vi "Tx Status to DBLs.vi"(3 "TxStatus":T1) -> (1 "TxStatusDBLs":dbl[](array[numeric]))   [LabVIEW 2020, in "AIM ARINC 664 Engine.lvlib" / "Implementation.lvlib" / "Tx Generic Execution Unit.lvclass"]
uses:
  Tx Generic Execution Unit.lvclass
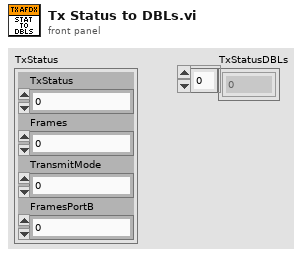
[diagram p1: front panel]
types:
  T1 = cluster{"TxStatus":u32, "Frames":u32, "TransmitMode":u32, "FramesPortB":u32}
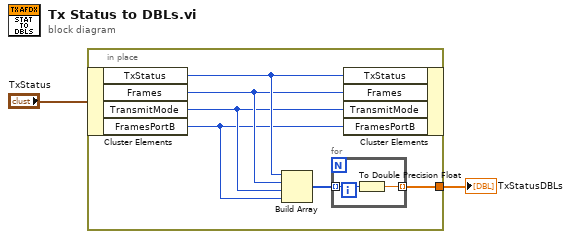
[diagram p0: block diagram]
diagram:
  n1 = in-place {
    in-place-border: [w3] -> w2
    n2 = in-place-cluster #1("TxStatus") -> ("TxStatus"=w8:u32, "Frames"=w7:u32, "TransmitMode"=w6:u32, "FramesPortB"=w5:u32)
    n3 = Build Array(w8, w7, w6, w5) -> (w4:u32[])
    n4 = for {
      tunnel: w4 -> [w10] mode=indexing
      tunnel: [w9] -> w3 mode=indexing
      n5 = To Double Precision Float(number=w10) -> (double precision float=w9:dbl)
    }
    n6 = in-place-cluster #1("TxStatus"=w8, "Frames"=w7, "TransmitMode"=w6, "FramesPortB"=w5) -> ()  [unwired: 1 out]
  }
  "TxStatusDBLs" <- w2
